vi "2D-Array sortieren.vi"(5 "Suchvorgabe":T1, 7 "Richtung":enum16{"v", "^"}(ring), 9 "2D-String-Array_in":string[][](array[string])=[["45245,25", "Hallo", "Eier"], ["45245,36", "Ballo", "Mehl"], ["45245,84", "Lallo", "Zucker"], ["245", "Trallo", "Salz"], ["45", "Knallo", "Bier"]]) -> (1 "2D-String-Array_nach Spalte 0 sortiert":string[][](array[string]))   [LabVIEW 2020, in "allgemeine Sub-VIs.lvlib"]
uses:
  allgemeine Sub-VIs.lvlib
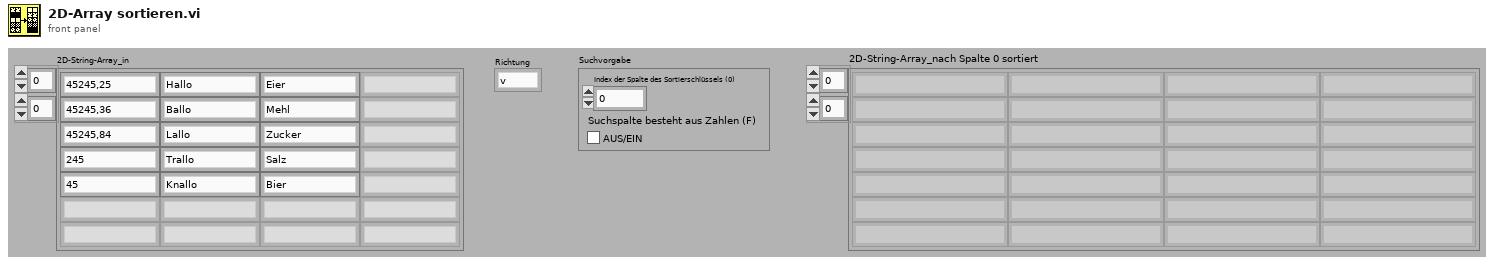
[diagram p1: front panel]
types:
  T1 = cluster{"Index der Spalte des Sortierschlüssels (0)":i32, "Suchspalte besteht aus Zahlen (F)":bool}
  T2 = cluster{"2D-String-Array_in[0]":string, "2D-String-Array_in[1]":string, "2D-String-Array_in[2]":string, "2D-String-Array_in[3]":string, "2D-String-Array_in[4]":string, "2D-String-Array_in[5]":string, "2D-String-Array_in[6]":string, "2D-String-Array_in[7]":string, "2D-String-Array_in[8]":string, "2D-String-Array_in[9]":string, "2D-String-Array_in[10]":string, "2D-String-Array_in[11]":string, "2D-String-Array_in[12]":string, "2D-String-Array_in[13]":string, "2D-String-Array_in[14]":string, "2D-String-Array_in[15]":string, "2D-String-Array_in[16]":string, "2D-String-Array_in[17]":string, "2D-String-Array_in[18]":string, "2D-String-Array_in[19]":string, "2D-String-Array_in[20]":string, "2D-String-Array_in[21]":string, "2D-String-Array_in[22]":string, "2D-String-Array_in[23]":string, "2D-String-Array_in[24]":string, "2D-String-Array_in[25]":string, "2D-String-Array_in[26]":string, "2D-String-Array_in[27]":string, "2D-String-Array_in[28]":string, "2D-String-Array_in[29]":string, "2D-String-Array_in[30]":string, "2D-String-Array_in[31]":string, "2D-String-Array_in[32]":string, "2D-String-Array_in[33]":string, "2D-String-Array_in[34]":string, "2D-String-Array_in[35]":string, "2D-String-Array_in[36]":string, "2D-String-Array_in[37]":string, "2D-String-Array_in[38]":string, "2D-String-Array_in[39]":string, "2D-String-Array_in[40]":string, "2D-String-Array_in[41]":string, "2D-String-Array_in[42]":string, "2D-String-Array_in[43]":string, "2D-String-Array_in[44]":string, "2D-String-Array_in[45]":string, "2D-String-Array_in[46]":string, "2D-String-Array_in[47]":string, "2D-String-Array_in[48]":string, "2D-String-Array_in[49]":string, "2D-String-Array_in[50]":string, "2D-String-Array_in[51]":string, "2D-String-Array_in[52]":string, "2D-String-Array_in[53]":string, "2D-String-Array_in[54]":string, "2D-String-Array_in[55]":string, "2D-String-Array_in[56]":string, "2D-String-Array_in[57]":string, "2D-String-Array_in[58]":string, "2D-String-Array_in[59]":string, "2D-String-Array_in[60]":string, "2D-String-Array_in[61]":string, "2D-String-Array_in[62]":string, "2D-String-Array_in[63]":string, "2D-String-Array_in[64]":string, "2D-String-Array_in[65]":string, "2D-String-Array_in[66]":string, "2D-String-Array_in[67]":string, "2D-String-Array_in[68]":string, "2D-String-Array_in[69]":string, "2D-String-Array_in[70]":string, "2D-String-Array_in[71]":string, "2D-String-Array_in[72]":string, "2D-String-Array_in[73]":string, "2D-String-Array_in[74]":string, "2D-String-Array_in[75]":string, "2D-String-Array_in[76]":string, "2D-String-Array_in[77]":string, "2D-String-Array_in[78]":string, "2D-String-Array_in[79]":string, "2D-String-Array_in[80]":string, "2D-String-Array_in[81]":string, "2D-String-Array_in[82]":string, "2D-String-Array_in[83]":string, "2D-String-Array_in[84]":string, "2D-String-Array_in[85]":string, "2D-String-Array_in[86]":string, "2D-String-Array_in[87]":string, "2D-String-Array_in[88]":string, "2D-String-Array_in[89]":string, "2D-String-Array_in[90]":string, "2D-String-Array_in[91]":string, "2D-String-Array_in[92]":string, "2D-String-Array_in[93]":string, "2D-String-Array_in[94]":string, "2D-String-Array_in[95]":string, "2D-String-Array_in[96]":string, "2D-String-Array_in[97]":string, "2D-String-Array_in[98]":string, "2D-String-Array_in[99]":string}
  T3 = cluster{dbl, "2D-String-Array_in":cluster{"2D-String-Array_in[0]":string, "2D-String-Array_in[1]":string, "2D-String-Array_in[2]":string, "2D-String-Array_in[3]":string, "2D-String-Array_in[4]":string, "2D-String-Array_in[5]":string, "2D-String-Array_in[6]":string, "2D-String-Array_in[7]":string, "2D-String-Array_in[8]":string, "2D-String-Array_in[9]":string, "2D-String-Array_in[10]":string, "2D-String-Array_in[11]":string, "2D-String-Array_in[12]":string, "2D-String-Array_in[13]":string, "2D-String-Array_in[14]":string, "2D-String-Array_in[15]":string, "2D-String-Array_in[16]":string, "2D-String-Array_in[17]":string, "2D-String-Array_in[18]":string, "2D-String-Array_in[19]":string, "2D-String-Array_in[20]":string, "2D-String-Array_in[21]":string, "2D-String-Array_in[22]":string, "2D-String-Array_in[23]":string, "2D-String-Array_in[24]":string, "2D-String-Array_in[25]":string, "2D-String-Array_in[26]":string, "2D-String-Array_in[27]":string, "2D-String-Array_in[28]":string, "2D-String-Array_in[29]":string, "2D-String-Array_in[30]":string, "2D-String-Array_in[31]":string, "2D-String-Array_in[32]":string, "2D-String-Array_in[33]":string, "2D-String-Array_in[34]":string, "2D-String-Array_in[35]":string, "2D-String-Array_in[36]":string, "2D-String-Array_in[37]":string, "2D-String-Array_in[38]":string, "2D-String-Array_in[39]":string, "2D-String-Array_in[40]":string, "2D-String-Array_in[41]":string, "2D-String-Array_in[42]":string, "2D-String-Array_in[43]":string, "2D-String-Array_in[44]":string, "2D-String-Array_in[45]":string, "2D-String-Array_in[46]":string, "2D-String-Array_in[47]":string, "2D-String-Array_in[48]":string, "2D-String-Array_in[49]":string, "2D-String-Array_in[50]":string, "2D-String-Array_in[51]":string, "2D-String-Array_in[52]":string, "2D-String-Array_in[53]":string, "2D-String-Array_in[54]":string, "2D-String-Array_in[55]":string, "2D-String-Array_in[56]":string, "2D-String-Array_in[57]":string, "2D-String-Array_in[58]":string, "2D-String-Array_in[59]":string, "2D-String-Array_in[60]":string, "2D-String-Array_in[61]":string, "2D-String-Array_in[62]":string, "2D-String-Array_in[63]":string, "2D-String-Array_in[64]":string, "2D-String-Array_in[65]":string, "2D-String-Array_in[66]":string, "2D-String-Array_in[67]":string, "2D-String-Array_in[68]":string, "2D-String-Array_in[69]":string, "2D-String-Array_in[70]":string, "2D-String-Array_in[71]":string, "2D-String-Array_in[72]":string, "2D-String-Array_in[73]":string, "2D-String-Array_in[74]":string, "2D-String-Array_in[75]":string, "2D-String-Array_in[76]":string, "2D-String-Array_in[77]":string, "2D-String-Array_in[78]":string, "2D-String-Array_in[79]":string, "2D-String-Array_in[80]":string, "2D-String-Array_in[81]":string, "2D-String-Array_in[82]":string, "2D-String-Array_in[83]":string, "2D-String-Array_in[84]":string, "2D-String-Array_in[85]":string, "2D-String-Array_in[86]":string, "2D-String-Array_in[87]":string, "2D-String-Array_in[88]":string, "2D-String-Array_in[89]":string, "2D-String-Array_in[90]":string, "2D-String-Array_in[91]":string, "2D-String-Array_in[92]":string, "2D-String-Array_in[93]":string, "2D-String-Array_in[94]":string, "2D-String-Array_in[95]":string, "2D-String-Array_in[96]":string, "2D-String-Array_in[97]":string, "2D-String-Array_in[98]":string, "2D-String-Array_in[99]":string}}
  T4 = cluster{dbl, "2D-String-Array_in":cluster{"2D-String-Array_in[0]":string, "2D-String-Array_in[1]":string, "2D-String-Array_in[2]":string, "2D-String-Array_in[3]":string, "2D-String-Array_in[4]":string, "2D-String-Array_in[5]":string, "2D-String-Array_in[6]":string, "2D-String-Array_in[7]":string, "2D-String-Array_in[8]":string, "2D-String-Array_in[9]":string, "2D-String-Array_in[10]":string, "2D-String-Array_in[11]":string, "2D-String-Array_in[12]":string, "2D-String-Array_in[13]":string, "2D-String-Array_in[14]":string, "2D-String-Array_in[15]":string, "2D-String-Array_in[16]":string, "2D-String-Array_in[17]":string, "2D-String-Array_in[18]":string, "2D-String-Array_in[19]":string, "2D-String-Array_in[20]":string, "2D-String-Array_in[21]":string, "2D-String-Array_in[22]":string, "2D-String-Array_in[23]":string, "2D-String-Array_in[24]":string, "2D-String-Array_in[25]":string, "2D-String-Array_in[26]":string, "2D-String-Array_in[27]":string, "2D-String-Array_in[28]":string, "2D-String-Array_in[29]":string, "2D-String-Array_in[30]":string, "2D-String-Array_in[31]":string, "2D-String-Array_in[32]":string, "2D-String-Array_in[33]":string, "2D-String-Array_in[34]":string, "2D-String-Array_in[35]":string, "2D-String-Array_in[36]":string, "2D-String-Array_in[37]":string, "2D-String-Array_in[38]":string, "2D-String-Array_in[39]":string, "2D-String-Array_in[40]":string, "2D-String-Array_in[41]":string, "2D-String-Array_in[42]":string, "2D-String-Array_in[43]":string, "2D-String-Array_in[44]":string, "2D-String-Array_in[45]":string, "2D-String-Array_in[46]":string, "2D-String-Array_in[47]":string, "2D-String-Array_in[48]":string, "2D-String-Array_in[49]":string, "2D-String-Array_in[50]":string, "2D-String-Array_in[51]":string, "2D-String-Array_in[52]":string, "2D-String-Array_in[53]":string, "2D-String-Array_in[54]":string, "2D-String-Array_in[55]":string, "2D-String-Array_in[56]":string, "2D-String-Array_in[57]":string, "2D-String-Array_in[58]":string, "2D-String-Array_in[59]":string, "2D-String-Array_in[60]":string, "2D-String-Array_in[61]":string, "2D-String-Array_in[62]":string, "2D-String-Array_in[63]":string, "2D-String-Array_in[64]":string, "2D-String-Array_in[65]":string, "2D-String-Array_in[66]":string, "2D-String-Array_in[67]":string, "2D-String-Array_in[68]":string, "2D-String-Array_in[69]":string, "2D-String-Array_in[70]":string, "2D-String-Array_in[71]":string, "2D-String-Array_in[72]":string, "2D-String-Array_in[73]":string, "2D-String-Array_in[74]":string, "2D-String-Array_in[75]":string, "2D-String-Array_in[76]":string, "2D-String-Array_in[77]":string, "2D-String-Array_in[78]":string, "2D-String-Array_in[79]":string, "2D-String-Array_in[80]":string, "2D-String-Array_in[81]":string, "2D-String-Array_in[82]":string, "2D-String-Array_in[83]":string, "2D-String-Array_in[84]":string, "2D-String-Array_in[85]":string, "2D-String-Array_in[86]":string, "2D-String-Array_in[87]":string, "2D-String-Array_in[88]":string, "2D-String-Array_in[89]":string, "2D-String-Array_in[90]":string, "2D-String-Array_in[91]":string, "2D-String-Array_in[92]":string, "2D-String-Array_in[93]":string, "2D-String-Array_in[94]":string, "2D-String-Array_in[95]":string, "2D-String-Array_in[96]":string, "2D-String-Array_in[97]":string, "2D-String-Array_in[98]":string, "2D-String-Array_in[99]":string}}[]
  T5 = cluster{"2D-String-Array_in[0]":string, "2D-String-Array_in[1]":string, "2D-String-Array_in[2]":string, "2D-String-Array_in[3]":string, "2D-String-Array_in[4]":string, "2D-String-Array_in[5]":string, "2D-String-Array_in[6]":string, "2D-String-Array_in[7]":string, "2D-String-Array_in[8]":string, "2D-String-Array_in[9]":string, "2D-String-Array_in[10]":string, "2D-String-Array_in[11]":string, "2D-String-Array_in[12]":string, "2D-String-Array_in[13]":string, "2D-String-Array_in[14]":string, "2D-String-Array_in[15]":string, "2D-String-Array_in[16]":string, "2D-String-Array_in[17]":string, "2D-String-Array_in[18]":string, "2D-String-Array_in[19]":string, "2D-String-Array_in[20]":string, "2D-String-Array_in[21]":string, "2D-String-Array_in[22]":string, "2D-String-Array_in[23]":string, "2D-String-Array_in[24]":string, "2D-String-Array_in[25]":string, "2D-String-Array_in[26]":string, "2D-String-Array_in[27]":string, "2D-String-Array_in[28]":string, "2D-String-Array_in[29]":string, "2D-String-Array_in[30]":string, "2D-String-Array_in[31]":string, "2D-String-Array_in[32]":string, "2D-String-Array_in[33]":string, "2D-String-Array_in[34]":string, "2D-String-Array_in[35]":string, "2D-String-Array_in[36]":string, "2D-String-Array_in[37]":string, "2D-String-Array_in[38]":string, "2D-String-Array_in[39]":string, "2D-String-Array_in[40]":string, "2D-String-Array_in[41]":string, "2D-String-Array_in[42]":string, "2D-String-Array_in[43]":string, "2D-String-Array_in[44]":string, "2D-String-Array_in[45]":string, "2D-String-Array_in[46]":string, "2D-String-Array_in[47]":string, "2D-String-Array_in[48]":string, "2D-String-Array_in[49]":string, "2D-String-Array_in[50]":string, "2D-String-Array_in[51]":string, "2D-String-Array_in[52]":string, "2D-String-Array_in[53]":string, "2D-String-Array_in[54]":string, "2D-String-Array_in[55]":string, "2D-String-Array_in[56]":string, "2D-String-Array_in[57]":string, "2D-String-Array_in[58]":string, "2D-String-Array_in[59]":string, "2D-String-Array_in[60]":string, "2D-String-Array_in[61]":string, "2D-String-Array_in[62]":string, "2D-String-Array_in[63]":string, "2D-String-Array_in[64]":string, "2D-String-Array_in[65]":string, "2D-String-Array_in[66]":string, "2D-String-Array_in[67]":string, "2D-String-Array_in[68]":string, "2D-String-Array_in[69]":string, "2D-String-Array_in[70]":string, "2D-String-Array_in[71]":string, "2D-String-Array_in[72]":string, "2D-String-Array_in[73]":string, "2D-String-Array_in[74]":string, "2D-String-Array_in[75]":string, "2D-String-Array_in[76]":string, "2D-String-Array_in[77]":string, "2D-String-Array_in[78]":string, "2D-String-Array_in[79]":string, "2D-String-Array_in[80]":string, "2D-String-Array_in[81]":string, "2D-String-Array_in[82]":string, "2D-String-Array_in[83]":string, "2D-String-Array_in[84]":string, "2D-String-Array_in[85]":string, "2D-String-Array_in[86]":string, "2D-String-Array_in[87]":string, "2D-String-Array_in[88]":string, "2D-String-Array_in[89]":string, "2D-String-Array_in[90]":string, "2D-String-Array_in[91]":string, "2D-String-Array_in[92]":string, "2D-String-Array_in[93]":string, "2D-String-Array_in[94]":string, "2D-String-Array_in[95]":string, "2D-String-Array_in[96]":string, "2D-String-Array_in[97]":string, "2D-String-Array_in[98]":string, "2D-String-Array_in[99]":string}[]
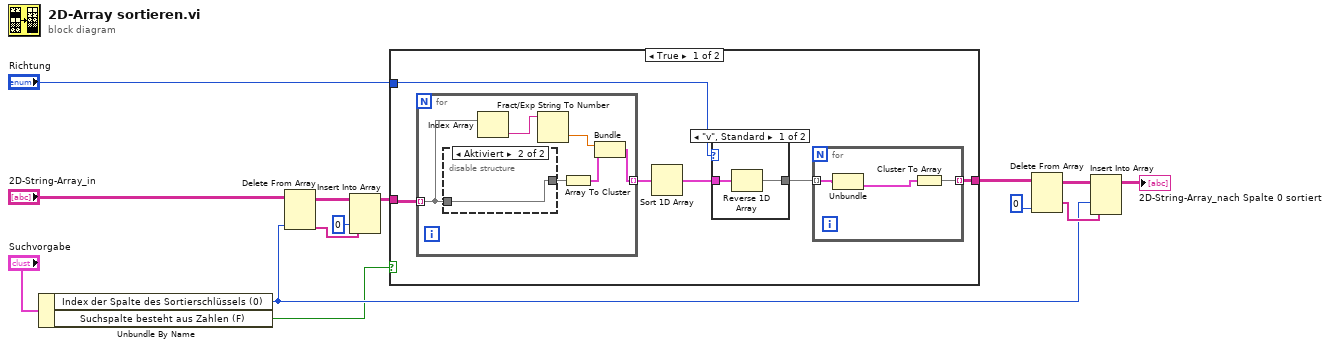
[diagram p0: block diagram]
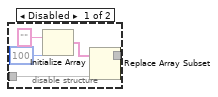
[diagram p3: hidden frame]
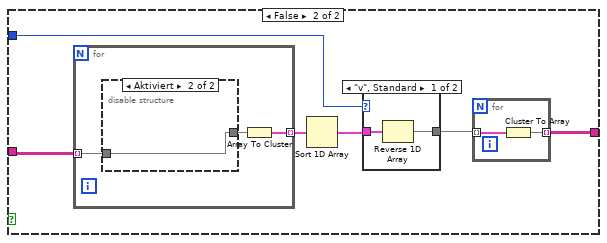
[diagram p4: hidden frame]
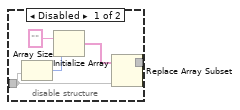
[diagram p6: hidden frame]
diagram:
  n1 = Unbundle By Name("Suchvorgabe") -> ("Index der Spalte des Sortierschlüssels (0)"=w4:i32, "Suchspalte besteht aus Zahlen (F)"=w3:bool)
  n2 = Delete From Array(array="2D-String-Array_in", index (col)=w4) -> (deleted portion=w6:string[], array with subset deleted=w14:string[][])  [unwired: 2 in]
  n3 = Insert Into Array(array=w14, index (col)=0 ("Deaktivierter Index (Spalte)"), new element=w6) -> (w12:string[][])  [unwired: 1 in]
  n4 = case shown="True" w3 {
    tunnel: w12 -> [w18 w39]
    tunnel: [w17 w43] -> w8
    tunnel: "Richtung" -> [w15 w40]
    frame True {
      n5 = for {
        tunnel: w18 -> [w28] mode=indexing
        tunnel: [w25] -> w20 mode=indexing
        n6 = disable-structure shown="Aktiviert" {
          disable-tunnel: [w31 w35] -> w29
          disable-tunnel: w28 -> [w30 w35]
          frame Disabled {
            n7 = Initialize Array("", 100 ("Dimensionsgröße")) -> (w32:string[])
            n8 = Replace Array Subset(array=w32, new element=w30) -> (w31:string[])  [unwired: 1 in]
          }
          frame Enabled {
          }
        }
        n9 = Index Array(array=w28) -> (element=w27:string)  [unwired: 1 in]
        n10 = Fract/Exp String To Number(string=w27) -> (number=w24:dbl)  [unwired: 3 in, 1 out]
        n11 = Array To Cluster(array=w29) -> (cluster=w26:T2)
        n12 = Bundle(w24, "2D-String-Array_in"=w26) -> (w25:T3)  [unwired: 1 in]
      }
      n13 = Sort 1D Array(array=w20) -> (sorted array=w19:T4)
      n14 = case shown="\"v\", Standard" w15 {
        tunnel: w19 -> [w22 w23]
        tunnel: [w21 w23] -> w16
        frame "v", Default {
          n15 = Reverse 1D Array(array=w22) -> (reversed array=w21:T4)
        }
        frame "^" {
        }
      }
      n16 = for {
        tunnel: w16 -> [w37] mode=indexing
        tunnel: [w38] -> w17 mode=indexing
        n17 = Unbundle(w37) -> ("2D-String-Array_in"=w36:T2)  [unwired: 1 out]
        n18 = Cluster To Array(cluster=w36) -> (array=w38:string[])
      }
    }
    frame False {
      n19 = for {
        tunnel: w39 -> [w48] mode=indexing
        tunnel: [w49] -> w44 mode=indexing
        n20 = disable-structure shown="Aktiviert" {
          disable-tunnel: [w53 w56] -> w50
          disable-tunnel: w48 -> [w52 w56]
          frame Disabled {
            n21 = Array Size(array=w52) -> (size(s)=w51:i32)
            n22 = Initialize Array("", w51) -> (w54:string[])
            n23 = Replace Array Subset(array=w54, new element=w52) -> (w53:string[])  [unwired: 1 in]
          }
          frame Enabled {
          }
        }
        n24 = Array To Cluster(array=w50) -> (cluster=w49:T2)
      }
      n25 = Sort 1D Array(array=w44) -> (sorted array=w42:T5)
      n26 = case shown="\"v\", Standard" w40 {
        tunnel: w42 -> [w46 w47]
        tunnel: [w45 w47] -> w41
        frame "v", Default {
          n27 = Reverse 1D Array(array=w46) -> (reversed array=w45:T5)
        }
        frame "^" {
        }
      }
      n28 = for {
        tunnel: w41 -> [w58] mode=indexing
        tunnel: [w57] -> w43 mode=indexing
        n29 = Cluster To Array(cluster=w58) -> (array=w57:string[])
      }
    }
  }
  n30 = Delete From Array(array=w8, index (col)=0 ("Deaktivierter Index (Spalte)")) -> (deleted portion=w11:string[], array with subset deleted=w10:string[][])  [unwired: 2 in]
  n31 = Insert Into Array(array=w10, index (col)=w4, new element=w11) -> (→"2D-String-Array_nach Spalte 0 sortiert":string[][])  [unwired: 1 in]
